vi "Nan_euclidean_distances.vi"(8 "error in":errorcluster caption="entrée d'erreur", 9 "Y":string[][](array[string]), 10 "X":string[][](array[string]), 11 "nan_euclidean_distances":T2={"squared"=FALSE, "missing_values"="nan", "copy"=TRUE}) -> (0 "error out":errorcluster caption="sortie d'erreur", 3 "Data":T1)   [LabVIEW 2020]
doc: "Calculate the euclidean distances in the presence of missing values.\n\nCompute the euclidean distance between each pair of samples in X and Y, where Y=X is assumed if Y=None. When calculating the distance between a pair of samples, this formulation ignores feature coordinates with a missing value in either sample and scales up the weight of the remaining coordinates:\n\ndist(x,y) = sqrt(weight * sq. distance from present coordinates) where, weight = Total # of coordinates / # of present coordinates\n\nIf all the coordinates are missing or if there are no common present coordinates then NaN is returned for that pair.\n\n\nParameters : \n\n- X : array-like, shape=(n_samples_1, n_features)\n\n- Y : array-like, shape=(n_samples_2, n_features)\nsquaredbool, default=False\nReturn squared Euclidean distances.\n\n- missing_values : np.nan or int, default=np.nan\nRepresentation of missing value\n\n- copy : boolean, default=True\nMake and use a deep copy of X and Y (if Y exists)\n\nReturns : \n\n- distances : array, shape (n_samples_1, n_samples_2)"
uses:
  Nan_euclidean_distances.lvclass
panel:
  out "Nan_euclidean_distances.lvclass":refnum<class "Nan_euclidean_distances.lvclass">
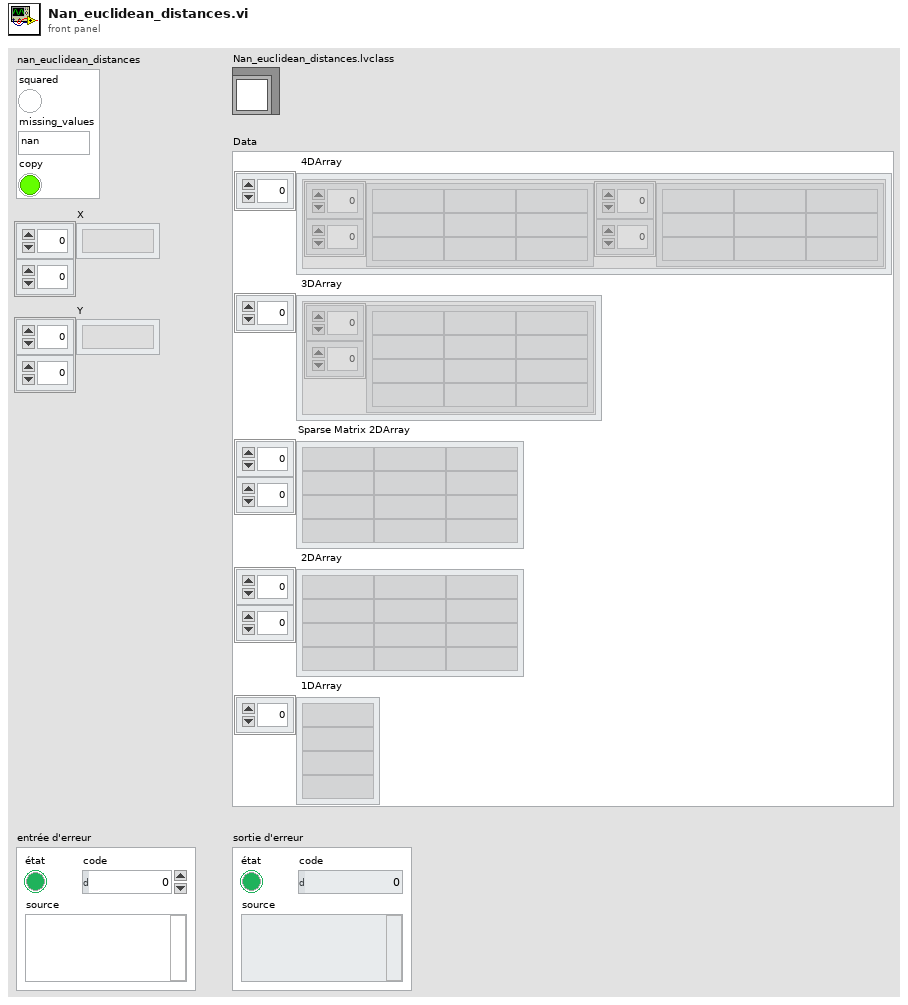
[diagram p1: front panel]
types:
  T1 = cluster{" 4DArray":cluster{"1":string[][], "2":string[][]}[], " 3DArray":cluster{"Tableau":string[][]}[], "Sparse Matrix 2DArray":string[][], " 2DArray":string[][], " 1DArray":string[]}
  T2 = cluster{"squared":bool, "missing_values":string, "copy":bool}
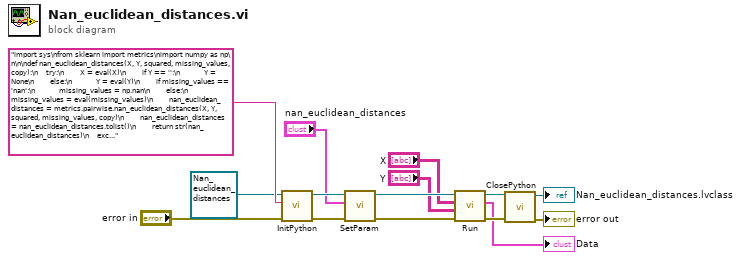
[diagram p0: block diagram]
diagram:
  n1 = call-dynamic "InitPython.vi"("error in (no error)"="error in", "Python Instruction"="import sys\nfrom sklearn import metrics\nimport numpy as np\n\n\ndef nan_euclidean_distances(X, Y, squared, missing_values, copy):\n    try:\n        X = eval(X)\n        if Y == '':\n            Y = None\n        else:\n            Y = eval(Y)\n        if missing_values == 'nan':\n            missing_values = np.nan\n        else:\n            missing_values = eval(missing_values)\n        nan_euclidean_distances = metrics.pairwise.nan_euclidean_distances(X, Y, squared, missing_values, copy)\n        nan_euclidean_distances = nan_euclidean_distances.tolist()\n        return str(nan_euclidean_distances)\n    except:\n        erreur = sys.exc_info()\n        typerr = u\"%s\" % (erreur[0])\n        typerr = typerr[typerr.find(\"'\")+1:typerr.rfind(\"'\")]\n        msgerr = u\"%s\" % (erreur[1])\n        message = str('/!\\\\ {0} : {1}'. format(typerr,msgerr))\n        return message", "Scikit-learn en entrée"=refnum<class "Nan_euclidean_distances.lvclass"> refnum ("Nan_euclidean_distances.lvclass")) -> ("error out"=w8:errorcluster, "Scikit-learn en sortie"=w10:refnum<class "Nan_euclidean_distances.lvclass">)  [unwired: 7 in]
  n2 = call-dynamic "SetParam.vi"("error in (no error)"=w8, "nan_euclidean_distances"="nan_euclidean_distances", "Nan_euclidean_distances.lvclass"=w10) -> ("error out"=w6:errorcluster, "Nan_euclidean_distances.lvclass"=w7:refnum<class "Nan_euclidean_distances.lvclass">)  [unwired: 7 in]
  n3 = call-dynamic "Run.vi"("error in (no error)"=w6, "Y"="Y", "X"="X", "Nan_euclidean_distances.lvclass"=w7) -> ("error out"=w13:errorcluster, "Data"=→"Data":T1, "Nan_euclidean_distances.lvclass"=w12:refnum<class "Nan_euclidean_distances.lvclass">)  [unwired: 5 in]
  n4 = call-dynamic "ClosePython.vi"("error in (no error)"=w13, "Scikit-learn en entrée"=w12) -> ("error out"=→"error out":errorcluster, "Scikit-learn en sortie"=→"Nan_euclidean_distances.lvclass":refnum<class "Nan_euclidean_distances.lvclass">)  [unwired: 8 in]
